vi "Query Tared Euler Angles.vi"(8 "error in":errorcluster {"code" format="%.0x"}, 11 "Session In":refnum<visa-resource-name>) -> (0 "error out":errorcluster {"code" format="%.0x"}, 2 "Euler Angles":dbl[](array[numeric]), 3 "Session Out":refnum<visa-resource-name>)   [LabVIEW 2012, in "YOST 3 Space.lvlib"]
uses:
  YOST 3 Space.lvlib
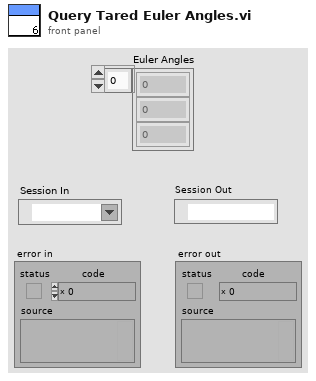
[diagram p1: front panel]
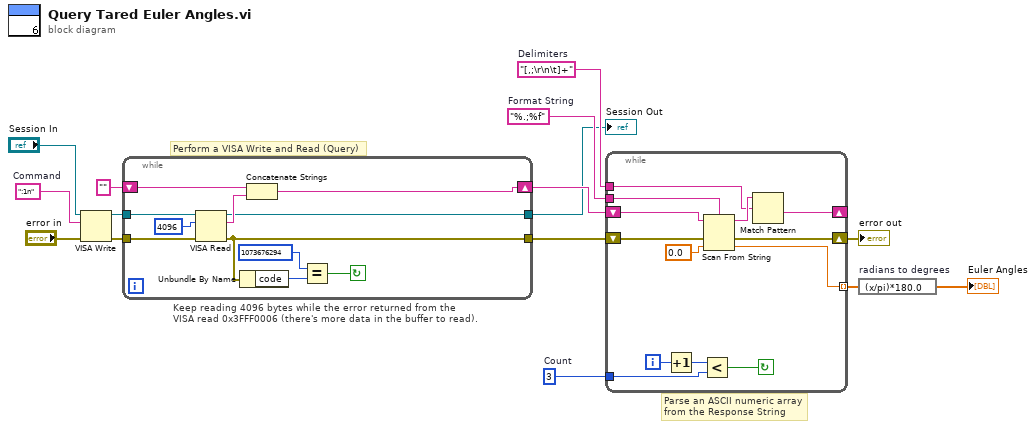
[diagram p0: block diagram]
diagram:
  w8 = "%.;%f"  # Format String
  w7 = "[,;\r\n\t]+"  # Delimiters
  w9 = 3  # Count
  w11 = ":1n"  # Command
  # "Parse an ASCII numeric array from the Response String"
  # "Perform a VISA Write and Read (Query)"
  # "Keep reading 4096 bytes while the error returned from the\nVISA read 0x3FFF0006 (there's more data in the buffer to read)."
  n1 = VISA Write(VISA resource name="Session In", write buffer=w11, error in (no error)="error in") -> (VISA resource name out=w15:refnum<visa-resource-name>, error out=w14:errorcluster)  [unwired: 1 out]
  n2 = while {
    tunnel: w15 -> [w23]
    shift-right: [w17] -> w10
    shift-left: "" -> [w22]
    tunnel: w14 -> [w20]
    tunnel: [w19] -> w13
    tunnel: [w16] -> w1
    stop <- w18 continue-if-true
    n3 = VISA Read(VISA resource name=w23, byte count=u32 4096 ("byte count (0)"), error in (no error)=w20) -> (VISA resource name out=w16:refnum<visa-resource-name>, read buffer=w21:string, error out=w19:errorcluster)  [unwired: 1 out]
    n4 = Unbundle By Name(w19) -> ("code"=w25:i32)
    n5 = Concatenate Strings(w22, w21) -> (w17:string)
    n6 = Equal?(x=1073676294, y=w25) -> (x = y?=w18:bool)
  }
  "Session Out" <- w1
  n7 = while {
    shift-right: [w29] -> _
    shift-left: w10 -> [w37]
    shift-right: [w28] -> w6
    shift-left: w13 -> [w36]
    tunnel: w9 -> [w33]
    tunnel: [w32] -> w5 mode=indexing
    tunnel: w8 -> [w31]
    tunnel: w7 -> [w27]
    i -> [w35]
    stop <- w38 continue-if-true
    n8 = Increment(x=w35) -> (x+1=w34:i32)
    n9 = Less?(x=w34, y=w33) -> (x < y?=w38:bool)
    n10 = Scan From String(format string=w31, input string=w37, error in=w36, default 1=0.0 ("Default Value 1")) -> (remaining string=w30:string, error out=w28:errorcluster, output 1=w32:dbl)  [unwired: 1 in, 1 out]
    n11 = Match Pattern(string=w30, regular expression=w27) -> (after substring=w29:string)  [unwired: 1 in, 3 out]
  }
  "error out" <- w6
  n12 = expression code="(x/pi)*180.0" "radians to degrees"(w5) -> (→"Euler Angles":dbl[])
